vi "Variant to Type.vi"(7 "Required? (F)":bool, 10 "Type In":T1, 11 "Value":variant) -> (2 "Type":T1)   [LabVIEW 2020, in "FlexBlock.xnode"]
uses:
  FlexBlock.xnode
  FlexBlocks/Type Descriptor.ctl
  FlexBlocks/Terminal Direction.ctl
  FlexBlocks/Value Mode.ctl
  FlexBlocks/Terminal State.ctl
  FlexBlocks/Special Terminal.ctl
  <vilib>/Utility/Data Type/NI_Data Type.lvlib
  FlexBlocks/FlexBlocks.lvlib
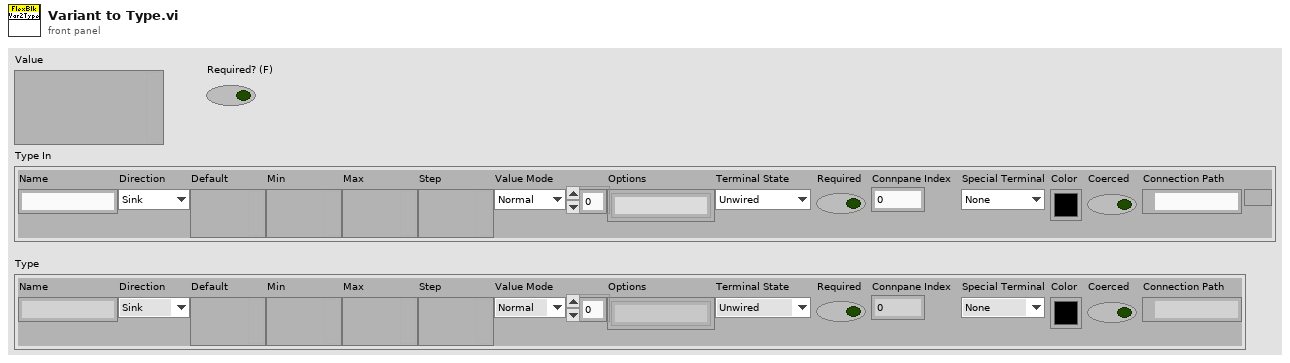
[diagram p1: front panel]
types:
  T1 = typedef "FlexBlocks.lvlib/Type Descriptor.ctl" = cluster{"Name":string, "Direction":T2, "Default":variant, "Min":variant, "Max":variant, "Step":variant, "Value Mode":T3, "Options":string[], "Terminal State":T4, "Required":bool, "Connpane Index":i32, "Special Terminal":T5, "Color":u32, "Coerced":bool, "Connection Path":path}
  T2 = typedef "FlexBlocks.lvlib/Terminal Direction.ctl" = enum16{"Sink", "Source"}
  T3 = typedef "FlexBlocks.lvlib/Value Mode.ctl" = enum16{"Normal", "Range", "Select"}
  T4 = typedef "FlexBlocks.lvlib/Terminal State.ctl" = enum16{"Unwired", "BadType", "BadRef", "Channel", "Value", "Control Ref"}
  T5 = typedef "FlexBlocks.lvlib/Special Terminal.ctl" = enum16{"None", "Action", "Init", "Tag", "State in", "State out", "Error"}
  T6 = typedef "NI_Data Type.lvlib/Data Type.ctl" = enum8{"Invalid Type", "Void", "I8", "I16", "I32", "I64", "U8", "U16", "U32", "U64", "Single Float", "Double Float", "Extended Float", "Single Complex", "Double Complex", "Extended Complex", "Enum U8", "Enum U16", "Enum U32", "Enum U64", "Single Float With Unit", "Double Float With Unit", "Extended Float With Unit", "Single Complex with Unit", "Double Complex with Unit", "Extended Complex with Unit", "Boolean", "String", "Path", "Picture", "Tag", "Array", "Cluster", "Variant", "LV Variant", "Waveform", "Timestamp", "Digital Waveform", "Digital Data", "ExpressData", "Refnum", "External Data", "VI", "Poly VI", "LabVIEW Class Instance", "Fixed Point", "Set Collection", "Map Collection"}
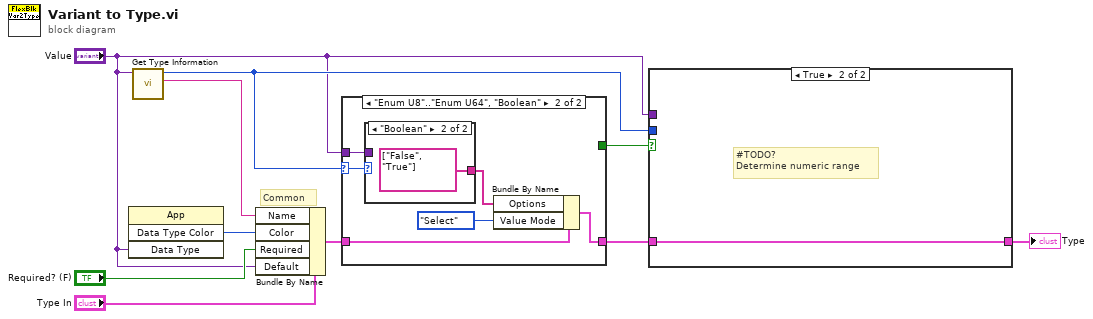
[diagram p0: block diagram]
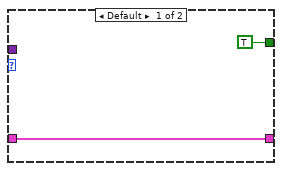
[diagram p3: hidden frame]
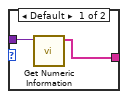
[diagram p4: hidden frame]
diagram:
  # "Common"
  n1 = invoke class="App" method="Data Type Color"("Data Type"="Value") -> ("Data Type Color"=w10:u32)  [unwired: 3 in, 3 out]
  n2 = call <vilib>:"Get Type Information.vi"("variant"="Value") -> ("name"=w9:string, "type"=w3:T6)  [unwired: 6 in, 3 out]
  n3 = Bundle By Name(cluster="Type In", "Name"=w9, "Color"=w10, "Required"="Required? (F)", "Default"="Value") -> (w7:T1)
  n4 = case shown="\"Enum U8\"..\"Enum U64\", \"Boolean\"" w3 {
    selector: w3 -> [_ w15]
    tunnel: w7 -> [w12 w18]
    tunnel: [w12 w17] -> w6
    tunnel: "Value" -> [_ w13]
    tunnel: [TRUE _] -> w5
    frame Default {
    }
    frame "Enum U8".."Enum U64", "Boolean" {
      n5 = case shown="\"Boolean\"" w15 {
        tunnel: [w19 string[] ["False", "True"]] -> w14
        tunnel: w13 -> [w20 _]
        frame Default {
          n6 = call <vilib>:"Get Numeric Information.vi"("variant"=w20) -> ("enum names"=w19:string[])  [unwired: 7 in, 3 out]
        }
        frame "Boolean" {
        }
      }
      n7 = Bundle By Name(cluster=w18, "Options"=w14, "Value Mode"=Value_Mode."Select") -> (w17:T1)
    }
  }
  n8 = case shown="True" w5 {
    tunnel: w6 -> [w22 w23]
    tunnel: [w22 w23] -> w4
    tunnel: "Value" -> [_ _]
    tunnel: w3 -> [_ _]
    frame False {
    }
    frame True {
      # "#TODO?\nDetermine numeric range"
    }
  }
  "Type" <- w4
